vi "DuplicateCells.vi"(6 "# Rows":i32, 8 "error in (no error)":errorcluster, 9 "Table CtlRef In":refnum<vi>, 10 "Cell Position":T1, 11 "SingleValMenuCol in":refnum<class "SingleValMenuCol.lvclass">) -> (0 "error out":errorcluster, 1 "Table CtlRef Out":refnum<vi>, 3 "SingleValMenuCol out":refnum<class "SingleValMenuCol.lvclass">)   [LabVIEW 2013, in "SingleValMenuCol.lvclass"]
doc: "Intended to be used as part of Insert Row(s) function, this method only copies formatting. Values can be more efficiently duplicated by row with array functions.\n\nThe funcitonality was made column-specific so that SingleVal can be handled appropriately."
uses:
  SingleValMenuCol.lvclass
  <vilib>/Utility/miscctls.llb/LVRowAndColumnTypeDef.ctl
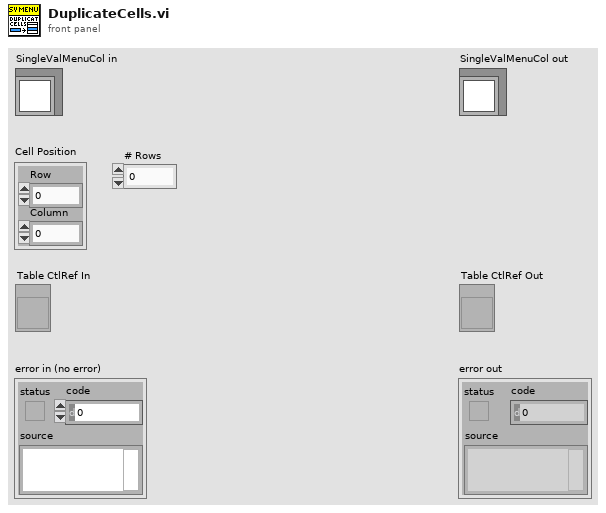
[diagram p1: front panel]
types:
  T1 = typedef "LVRowAndColumnTypeDef.ctl" = cluster{"Row":i32, "Column":i32}
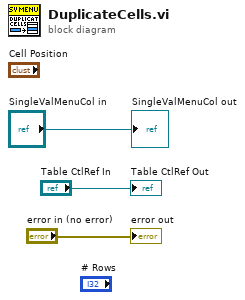
[diagram p0: block diagram]
diagram:
  "error out" <- "error in (no error)"
  "SingleValMenuCol out" <- "SingleValMenuCol in"
  "Table CtlRef Out" <- "Table CtlRef In"
